vi "WriteLogFiles.vi"(8 "error in (no error)":errorcluster, 11 "path":path) -> (0 "error out":errorcluster)   [LabVIEW 2017, in "USBDrive.lvlib"]
uses:
  <vilib>/addons/InsightCM/Devices/Shared/Common/USBDrive/USBDrive.lvlib
  <vilib>/addons/InsightCM/Utilities/GlobalConfiguration/GlobalConfiguration.lvlib
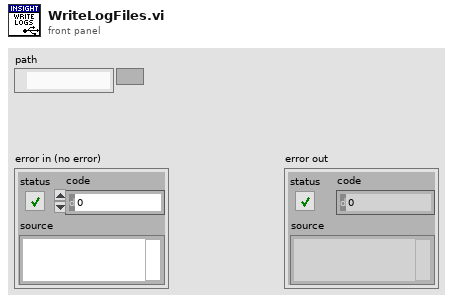
[diagram p1: front panel]
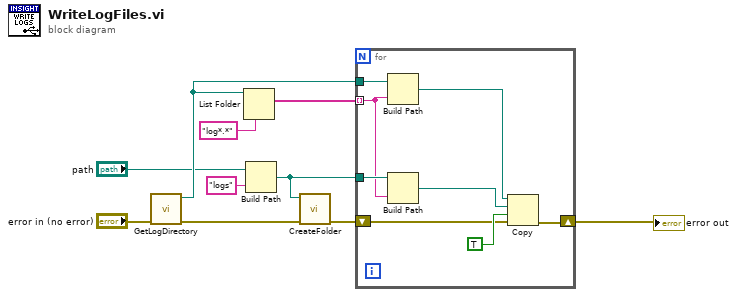
[diagram p0: block diagram]
diagram:
  n1 = call <vilib>:"GetLogDirectory.vi"("error in (no error)"="error in (no error)") -> ("error out"=w3:errorcluster, "log dir"=w6:path)  [unwired: 9 in]
  n2 = List Folder(path=w6, pattern="log*.*" ("name or relative path")) -> (filenames=w9:string[])  [unwired: 2 in, 3 out]
  n3 = Build Path(base path="path", name or relative path="logs") -> (appended path=w1:path)
  n4 = call <vilib>:"CreateFolder.vi"("error in (no error)"=w3, "folder"=w1) -> ("error out"=w2:errorcluster)  [unwired: 8 in, 1 out]
  n5 = for {
    tunnel: w6 -> [w18]
    tunnel: w9 -> [w15] mode=indexing
    tunnel: w1 -> [w16]
    shift-right: [w13] -> w8
    shift-left: w2 -> [w11]
    n6 = Build Path(base path=w18, name or relative path=w15) -> (appended path=w17:path)
    n7 = Build Path(base path=w16, name or relative path=w15) -> (appended path=w14:path)
    n8 = Copy(8:w11, 9:TRUE ("overwrite (F)"), 10:w14, 11:w17) -> (0:w13:errorcluster)  [unwired: 1 in, 2 out]
  }
  "error out" <- w8
